vi "Hang Tele-Op.vi"(9 "Buttons":bool[](array[boolean]), 10 "Axes":dbl[](array[numeric]), 11 "Driver Buttons":bool[](array[boolean])) -> ()   [LabVIEW 2019]
uses:
  <vilib>/Rock Robotics/WPI/Solenoid/WPI_SolenoidValue.ctl
  be246d07-8f40-4d14-8f8a-417157138aa0.vi
  aa87c3a5-c8b7-4379-aa0a-94ac4ae14cab.vi
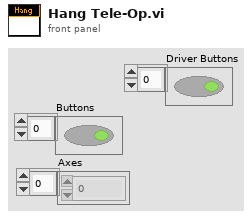
[diagram p1: front panel]
types:
  T1 = typedef "WPI_SolenoidValue.ctl" = enum16{"Off", "On", "Forward", "Reverse"}
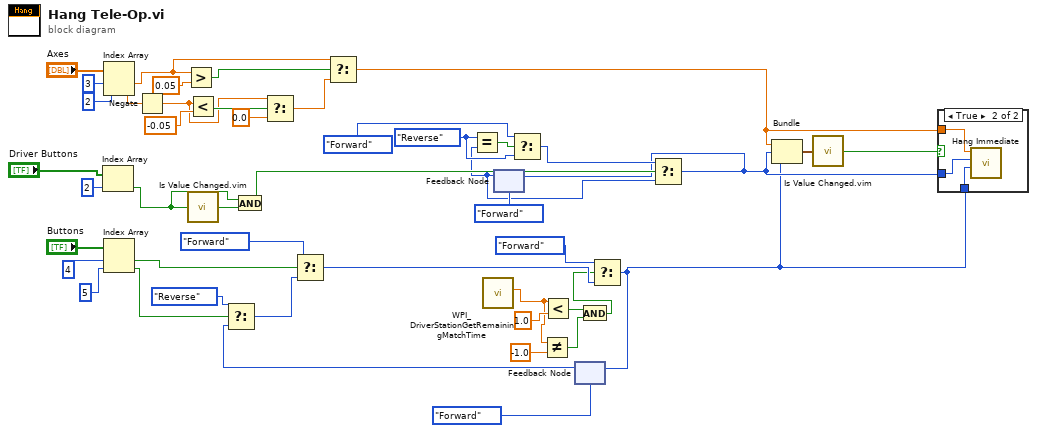
[diagram p0: block diagram]
diagram:
  w38 = WPI_SolenoidValue."Reverse" ("x")
  n1 = Index Array(array="Driver Buttons", index=2) -> (element=w18:bool)
  n2 = Index Array(array="Axes", index #1=3 ("index"), index #2=2 ("index")) -> (element #1=w25:dbl, element #2=w23:dbl)
  n3 = Index Array(array="Buttons", index #1=4 ("index"), index #2=5 ("index")) -> (element #1=w16:bool, element #2=w15:bool)
  n4 = Negate(x=w23) -> (-x=w22:dbl)
  n5 = Greater?(x=w25, y=0.05) -> (0:w26:bool)
  n6 = Less?(x=w22, y=-0.05) -> (x < y?=w28:bool)
  n7 = call "Is Value Changed.vim"("value"=w18) -> ("changed or first call?"=w43:bool)
  n8 = And(x=w18, y=w43) -> (x .and. y?=w41:bool)
  n9 = Select(t=w22, s=w28, f=0.0) -> (s? t:f=w29:dbl)
  n10 = Select(t=w25, s=w26, f=w29) -> (s? t:f=w24:dbl)
  n11 = call <vilib>:"WPI_DriverStationGetRemainingMatchTime.vi"() -> ("Match Time(s)"=w4:sgl)  [unwired: 10 in, 1 out]
  n12 = feedback #1(WPI_SolenoidValue."Forward" ("Angle")) -> (w36:T1)
  n13 = Equal?(x=w38, y=w36) -> (x = y?=w40:bool)
  n14 = Select(t=WPI_SolenoidValue."Forward" ("Angle"), s=w40, f=w38) -> (s? t:f=w37:T1)
  n15 = Not Equal?(x=w4, y=sgl -1.0) -> (x != y?=w2:bool)
  n16 = Less?(x=w4, y=sgl 1.0) -> (x < y?=w5:bool)
  n17 = feedback #2(WPI_SolenoidValue."Forward" ("f")) -> (w11:T1)
  n18 = Select(t=WPI_SolenoidValue."Reverse" ("f"), s=w15, f=w11) -> (s? t:f=w12:T1)
  n19 = Select(t=WPI_SolenoidValue."Forward" ("Angle"), s=w16, f=w12) -> (s? t:f=w8:T1)
  n20 = And(x=w5, y=w2) -> (x .and. y?=w1:bool)
  n21 = Select(t=WPI_SolenoidValue."Forward", s=w1, f=w8) -> (s? t:f=w6:T1)
  n22 = feedback-in #2(w6) -> ()
  n23 = Select(t=w37, s=w41, f=w36) -> (s? t:f=w35:T1)
  n24 = feedback-in #1(w35) -> ()
  n25 = Bundle("f"=w24, "Angle"=w35, "f"=w6) -> (w45:cluster{"f":dbl, "Angle":T1, "f":T1})  [unwired: 1 in]
  n26 = call "Is Value Changed.vim"("value"=w45) -> ("changed or first call?"=w44:bool)
  n27 = case shown="True" w44 {
    tunnel: w35 -> [_ w49]
    tunnel: w24 -> [_ w48]
    tunnel: w6 -> [_ w47]
    frame False {
    }
    frame True {
      n28 = call "Hang Immediate.vi"("Ratchet"=w47, "Angle"=w49, "Setpoint"=w48) -> ()  [unwired: 9 in]
    }
  }
